vi "Setup.vi"(10 "Actor":refnum<class "Actor.lvclass">, 11 "Ex Event Actor in":refnum<class "Ex Event Actor.lvclass">) -> (3 "Ex Event Actor out":refnum<class "Ex Event Actor.lvclass">)   [LabVIEW 2021, in "Ex Event Actor.lvclass"]
uses:
  Ex Event Actor.lvclass
  Actor/Actor/Actor.lvclass
  Actor/Event Actor/Event Actor.lvclass
  Ex Event Actor.lvclass/Ex Event Actor.ctl
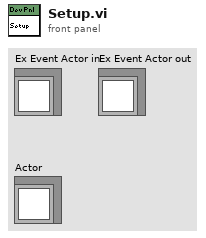
[diagram p1: front panel]
types:
  T1 = enum32{"Invalid", "Standard", "Closed", "Hidden", "Minimized", "Maximized"}
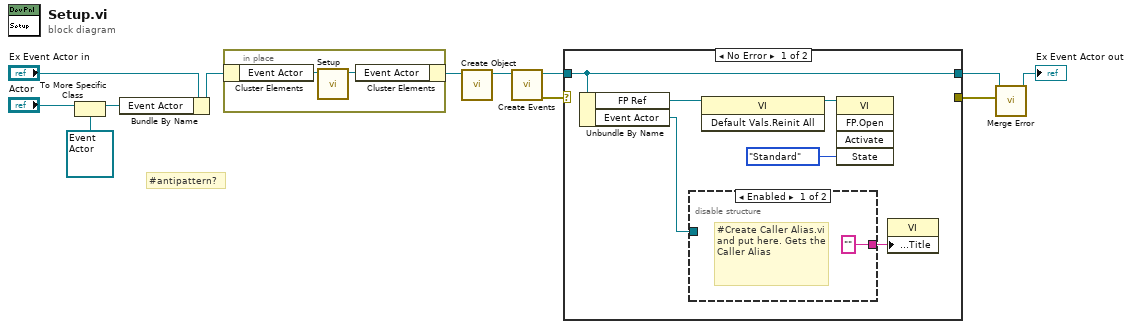
[diagram p0: block diagram]
diagram:
  # "#antipattern?"
  n1 = To More Specific Class(target class=refnum<class "Event Actor.lvclass"> refnum ("Event Actor.lvclass"), reference="Actor") -> (specific class reference=w2:refnum<class "Event Actor.lvclass">)  [unwired: 1 in, 1 out]
  n2 = Bundle By Name(cluster="Ex Event Actor in", "Event Actor"=w2) -> (w7:refnum<class "Ex Event Actor.lvclass">)
  n3 = in-place {
    n4 = in-place-cluster #1(w7) -> ("Event Actor"=w14:refnum<class "Event Actor.lvclass">)
    n5 = call-dynamic "Setup.vi"("Actor in"=w14) -> ("Actor out"=w13:refnum<class "Event Actor.lvclass">)  [unwired: 10 in]
    n6 = in-place-cluster #1("Event Actor"=w13) -> (w9:refnum<class "Ex Event Actor.lvclass">)
  }
  n7 = call "Create Object.vi"("Ex Event Actor in"=w9) -> ("Ex Event Actor out"=w5:refnum<class "Ex Event Actor.lvclass">)  [unwired: 10 in]
  n8 = call "Create Events.vi"("Ex Event Actor in"=w5) -> ("error out"=w3:errorcluster, "Ex Event Actor out"=w4:refnum<class "Ex Event Actor.lvclass">)  [unwired: 9 in]
  n9 = case shown="No Error" w3 {
    selector: w3 -> [_ w22]
    tunnel: w4 -> [w15 w23]
    tunnel: [w15 w23] -> w12
    tunnel: [_ w22] -> w11
    frame No Error {
      n10 = Unbundle By Name(w15) -> ("FP Ref"=w18:refnum<vi>, "Event Actor"=w16:refnum<class "Event Actor.lvclass">)
      n11 = disable-structure shown="Enabled" {
        disable-tunnel: ["" ("Front Panel Window:Title") _] -> w17
        disable-tunnel: w16 -> [_ _]
        frame Enabled {
          # "#Create Caller Alias.vi\nand put here. Gets the Caller Alias"
        }
        frame Disabled {
        }
      }
      n12 = invoke class="VI" method="Default Vals.Reinit All"(reference=w18) -> (reference out=w19:refnum<vi>)  [unwired: 2 in, 2 out]
      n13 = invoke class="VI" method="FP.Open"(reference=w19, "State"=T1."Standard") -> ()  [unwired: 3 in, 5 out]
      n14 = property class="VI"("Front Panel.Title"=w17) -> ()  [unwired: 2 in, 2 out]
    }
    frame Error {
    }
  }
  n15 = call-dynamic "Merge Error.vi"("Error"=w11, "Set Error in"=w12) -> ("Set Error out"=→"Ex Event Actor out":refnum<class "Ex Event Actor.lvclass">)  [unwired: 9 in]
